vi "客服端数据.vi"(0 "客P-主IP:P":string, 2 "数据输入":T1, 11 "报文最大量":u16=1200, 12 "枚举":T2(ring)) -> (14 "找不到键？":bool, 16 "数据获取":T1)   [LabVIEW 2019, in "MainPage.lvlib" / "MainPage.lvclass"]
uses:
  MainPage.lvclass
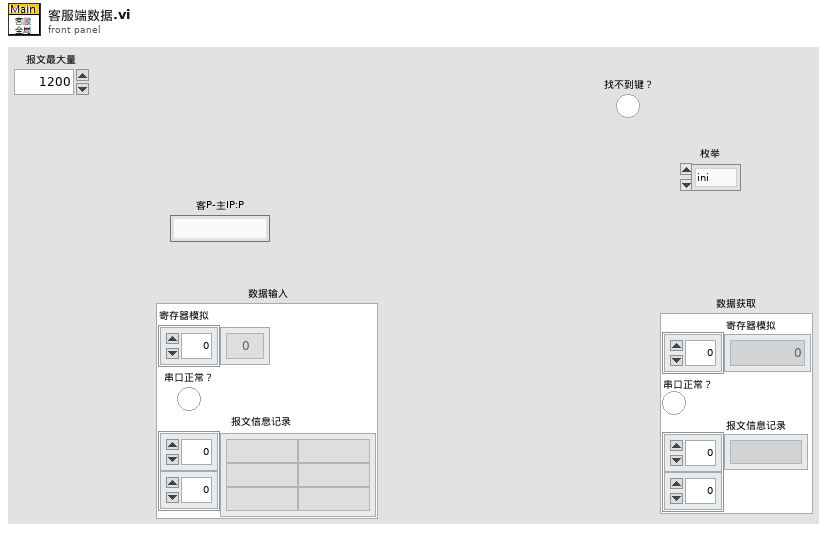
[diagram p1: front panel]
types:
  T1 = cluster{"寄存器模拟":u16[], "串口正常？":bool, "报文信息记录":string[][]}
  T2 = enum16{"ini", "增加记录", "读取记录", "更改寄存器值", "更改接口状态", "更改报文信息", "增加报文信息"}
  T3 = map{string, cluster{"寄存器模拟":u16[], "串口正常？":bool, "报文信息记录":string[][]}}
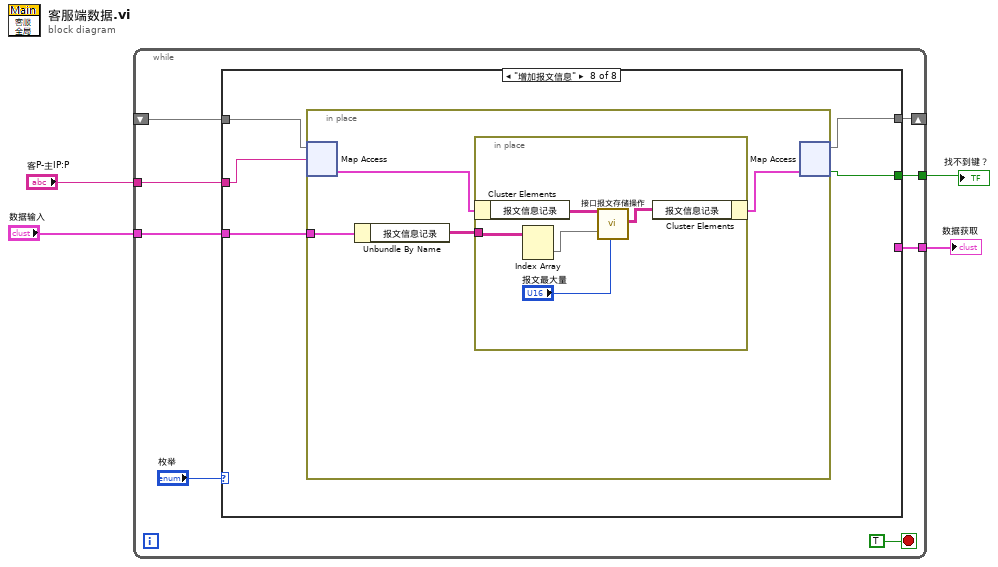
[diagram p0: block diagram]
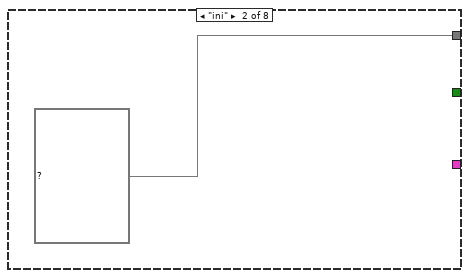
[diagram p3: hidden frame]
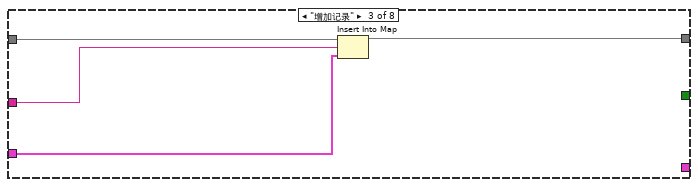
[diagram p4: hidden frame]
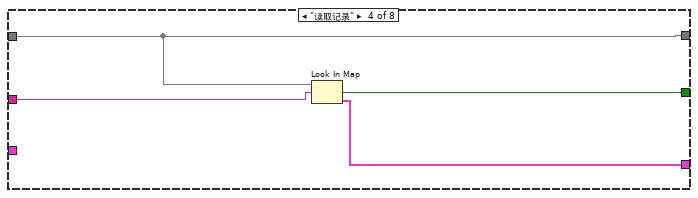
[diagram p5: hidden frame]
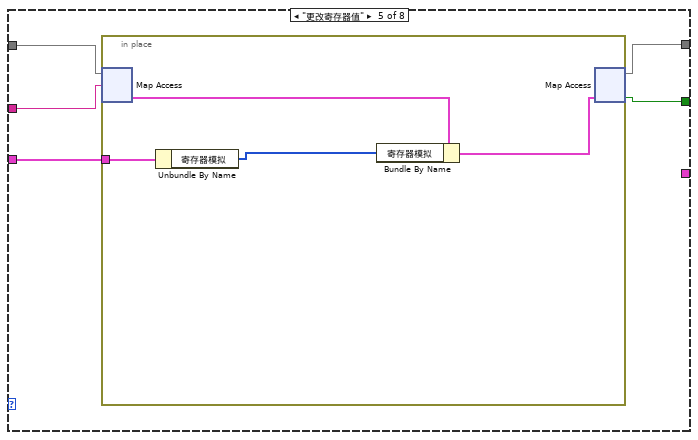
[diagram p6: hidden frame]
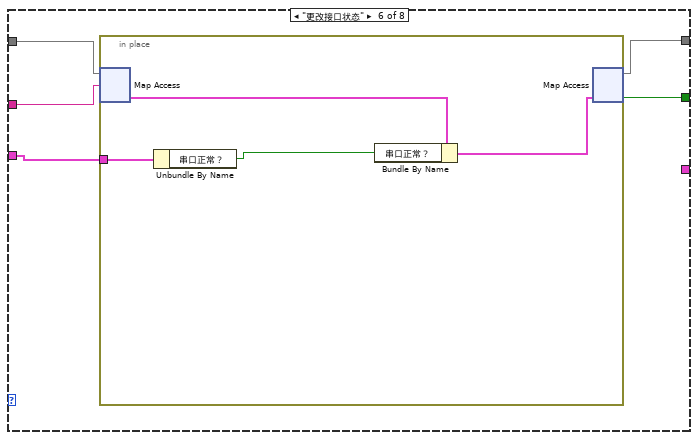
[diagram p7: hidden frame]
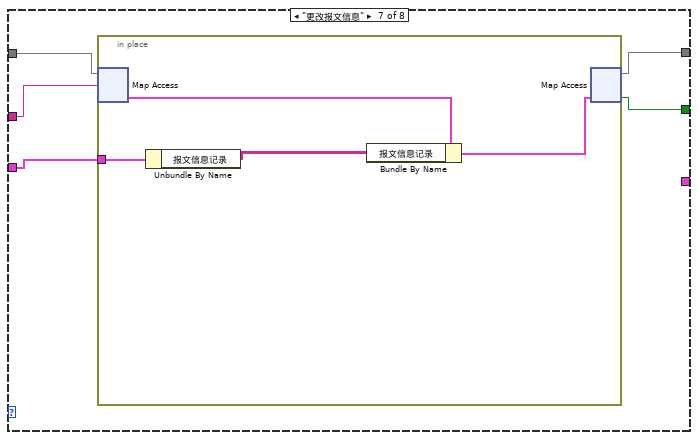
[diagram p8: hidden frame]
diagram:
  n1 = while {
    shift-right: [w11] -> _
    shift-left: _ -> [w10]
    tunnel: "客P-主IP:P" -> [w8]
    tunnel: "数据输入" -> [w7]
    tunnel: [w6] -> w2
    tunnel: [w5] -> w1
    stop <- TRUE stop-if-true
    n2 = case shown="\"增加报文信息\"" "枚举" {
      tunnel: [w13 T3 {} ("服务端记录") w17 w22 w24 w36 w42 w50] -> w11
      tunnel: w10 -> [w13 _ w18 w22 w27 w35 w45 w54]
      tunnel: w8 -> [_ _ w16 w21 w26 w33 w43 w52]
      tunnel: w7 -> [_ _ w15 _ w25 w34 w44 w53]
      tunnel: [_ _ _ w20 _ _ _ _] -> w6
      tunnel: [_ _ _ w19 w23 w32 w41 w51] -> w5
      frame Default {
      }
      frame "ini" {
      }
      frame "增加记录" {
        n3 = Insert Into Map(map in=w18, key=w16, value=w15) -> (map out=w17:T3)  [unwired: 2 out]
      }
      frame "读取记录" {
        n4 = Look In Map(map=w22, key=w21) -> (key not found?=w19:bool, value=w20:T1)  [unwired: 1 in]
      }
      frame "更改寄存器值" {
        n5 = in-place {
          in-place-border: w25 -> [w31]
          n6 = in-place-map #1(w27, w26) -> (w30:T1)  [unwired: 1 in, 1 out]
          n7 = Unbundle By Name(w31) -> ("寄存器模拟"=w29:u16[])
          n8 = Bundle By Name(cluster=w30, "寄存器模拟"=w29) -> (w28:T1)
          n9 = in-place-map #1(w28) -> (w24:T3, w23:bool)  [unwired: 1 in, 1 out]
        }
      }
      frame "更改接口状态" {
        n10 = in-place {
          in-place-border: w34 -> [w40]
          n11 = in-place-map #2(w35, w33) -> (w39:T1)  [unwired: 1 in, 1 out]
          n12 = Unbundle By Name(w40) -> ("串口正常？"=w38:bool)
          n13 = Bundle By Name(cluster=w39, "串口正常？"=w38) -> (w37:T1)
          n14 = in-place-map #2(w37) -> (w36:T3, w32:bool)  [unwired: 1 in, 1 out]
        }
      }
      frame "更改报文信息" {
        n15 = in-place {
          in-place-border: w44 -> [w49]
          n16 = in-place-map #3(w45, w43) -> (w48:T1)  [unwired: 1 in, 1 out]
          n17 = Unbundle By Name(w49) -> ("报文信息记录"=w47:string[][])
          n18 = Bundle By Name(cluster=w48, "报文信息记录"=w47) -> (w46:T1)
          n19 = in-place-map #3(w46) -> (w42:T3, w41:bool)  [unwired: 1 in, 1 out]
        }
      }
      frame "增加报文信息" {
        n20 = in-place {
          in-place-border: w53 -> [w58]
          n21 = in-place-map #4(w54, w52) -> (w57:T1)  [unwired: 1 in, 1 out]
          n22 = Unbundle By Name(w58) -> ("报文信息记录"=w56:string[][])
          n23 = in-place {
            in-place-border: w56 -> [w60]
            n24 = in-place-cluster #5(w57) -> ("报文信息记录"=w63:string[][])
            n25 = Index Array(array=w60) -> (element=w59:string[])  [unwired: 2 in]
            n26 = call "接口报文存储操作.vi"("原始记录"=w63, "报文信息"=w59, "报文最大量"="报文最大量") -> ("输出记录"=w62:string[][])  [unwired: 16 in]
            n27 = in-place-cluster #5("报文信息记录"=w62) -> (w55:T1)
          }
          n28 = in-place-map #4(w55) -> (w50:T3, w51:bool)  [unwired: 1 in, 1 out]
        }
      }
    }
  }
  "数据获取" <- w2
  "找不到键？" <- w1
